vi "getPayloadLength.vi"(11 "ControlPacket in":refnum<class "ControlPacket.lvclass">) -> (2 "Payload size":u32, 3 "ControlPacket out":refnum<class "ControlPacket.lvclass">)   [LabVIEW 2013, in "ControlPacket.lvclass"]
uses:
  ControlPacket.lvclass
  ControlPacket.lvclass/ControlPacket.ctl
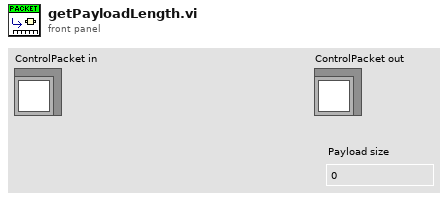
[diagram p1: front panel]
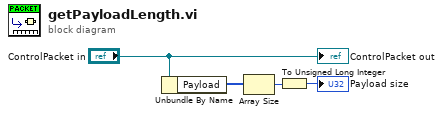
[diagram p0: block diagram]
diagram:
  n1 = Unbundle By Name("ControlPacket in") -> ("Payload"=w2:u8[])
  n2 = Array Size(array=w2) -> (size(s)=w4:i32)
  n3 = To Unsigned Long Integer(number=w4) -> (unsigned 32bit integer=→"Payload size":u32)
  "ControlPacket out" <- "ControlPacket in"
